vi "Get Sub Items.vi"(8 "error in (no error)":errorcluster, 11 "Type in":variant) -> (0 "error out":errorcluster, 2 "Sub Items":cluster{"Sub Items":T1[]}[](array[cluster]), 3 "Type out":variant)   [LabVIEW 2015, in "Read-Write-Signals.xnode"]
uses:
  Read-Write-Signals.xnode
  Read-Write-Signals Sub Item.ctl
  Read-Write-Signals Sub Item Type.ctl
  <vilib>/Utility/Data Type/NI_Data Type.lvlib
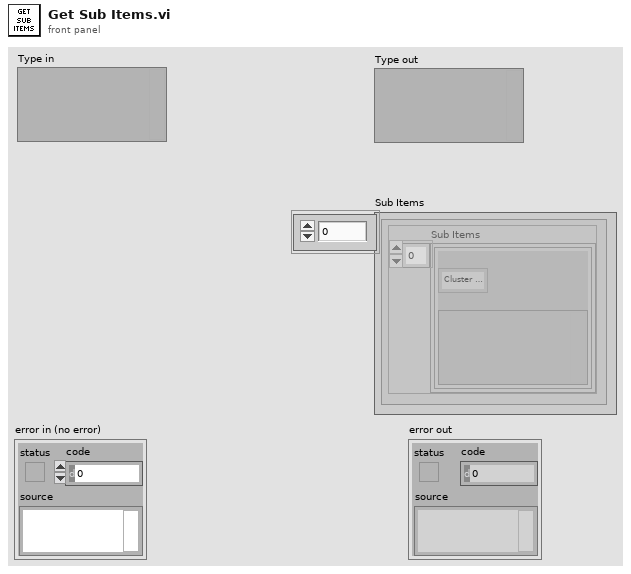
[diagram p1: front panel]
types:
  T1 = typedef "Read-Write-Signals Sub Item.ctl" = cluster{"Type":T2, "Value":variant}
  T2 = typedef "Read-Write-Signals Sub Item Type.ctl" = enum8{"Cluster Element", "Array Element", "Subarray"}
  T3 = typedef "NI_Data Type.lvlib/Data Type.ctl" = enum8{"Invalid Type", "Void", "I8", "I16", "I32", "I64", "U8", "U16", "U32", "U64", "Single Float", "Double Float", "Extended Float", "Single Complex", "Double Complex", "Extended Complex", "Enum U8", "Enum U16", "Enum U32", "Enum U64", "Single Float With Unit", "Double Float With Unit", "Extended Float With Unit", "Single Complex with Unit", "Double Complex with Unit", "Extended Complex with Unit", "Boolean", "String", "Path", "Picture", "Tag", "Array", "Cluster", "Variant", "LV Variant", "Waveform", "Timestamp", "Digital Waveform", "Digital Data", "ExpressData", "Refnum", "External Data", "VI", "Poly VI", "LabVIEW Class Instance", "Fixed Point"}
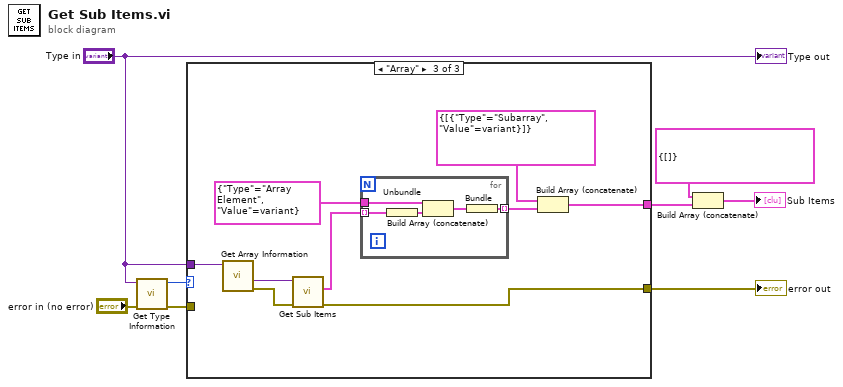
[diagram p0: block diagram]
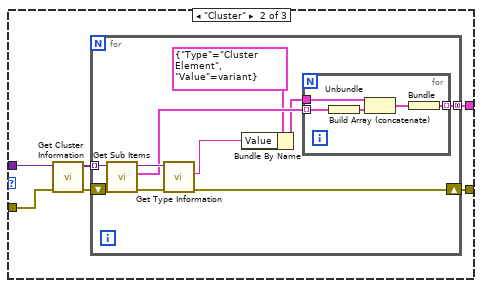
[diagram p3: hidden frame]
diagram:
  n1 = call <vilib>:"Get Type Information.vi"("error in (no error)"="error in (no error)", "Variant"="Type in") -> ("error out"=w6:errorcluster, "Type"=w8:T3)  [unwired: 5 in, 3 out]
  n2 = case shown="\"Array\"" w8 {
    tunnel: "Type in" -> [_ w15 w38]
    tunnel: w6 -> [w9 w14 _]
    tunnel: [_ w11 w31] -> w3
    tunnel: [w9 w10 w35] -> w4
    frame Default {
    }
    frame "Cluster" {
      n3 = call <vilib>:"Get Cluster Information.vi"("error in (no error)"=w14, "Variant"=w15) -> ("error out"=w12:errorcluster, "Cluster Elements"=w13:variant[])  [unwired: 8 in]
      n4 = for {
        tunnel: w13 -> [w25] mode=indexing
        tunnel: [w17] -> w11 mode=concatenating
        shift-right: [w16] -> w10
        shift-left: w12 -> [w24]
        n5 = call "Get Sub Items.vi"("error in (no error)"=w24, "Type in"=w25) -> ("error out"=w22:errorcluster, "Sub Items"=w21:cluster{"Sub Items":T1[]}[], "Type out"=w23:variant)  [unwired: 7 in]
        n6 = call <vilib>:"Get Type Information.vi"("error in (no error)"=w22, "Variant"=w23) -> ("error out"=w16:errorcluster, "Name"=w19:string)  [unwired: 5 in, 3 out]
        n7 = Bundle By Name(cluster=T1 {"Type"=enum."Cluster Element", "Value"=variant} ("Sub Items 2"), "Value"=w19) -> (w18:T1)
        n8 = for {
          tunnel: w21 -> [w30] mode=indexing
          tunnel: w18 -> [w28]
          tunnel: [w26] -> w17 mode=indexing
          n9 = Unbundle(w30) -> ("Sub Items"=w29:T1[])
          n10 = Build Array (concatenate)(w28, w29) -> (w27:T1[])
          n11 = Bundle(w27) -> (w26:cluster{T1[]})  [unwired: 1 in]
        }
      }
    }
    frame "Array" {
      n12 = call <vilib>:"Get Array Information.vi"("Variant"=w38) -> ("error out"=w36:errorcluster, "Array Element Data Type"=w37:variant)  [unwired: 7 in, 2 out]
      n13 = call "Get Sub Items.vi"("error in (no error)"=w36, "Type in"=w37) -> ("error out"=w35:errorcluster, "Sub Items"=w39:cluster{"Sub Items":T1[]}[])  [unwired: 7 in, 1 out]
      n14 = for {
        tunnel: w39 -> [w44] mode=indexing
        tunnel: T1 {"Type"=enum."Array Element", "Value"=variant} ("Sub Items 2") -> [w42]
        tunnel: [w40] -> w33 mode=indexing
        n15 = Unbundle(w44) -> ("Sub Items"=w43:T1[])
        n16 = Build Array (concatenate)(w42, w43) -> (w41:T1[])
        n17 = Bundle(w41) -> (w40:cluster{T1[]})  [unwired: 1 in]
      }
      n18 = Build Array (concatenate)(cluster{T1[]} {[{"Type"=enum."Subarray", "Value"=variant}]}, w33) -> (w31:cluster{T1[]}[])
    }
  }
  "error out" <- w4
  n19 = Build Array (concatenate)(cluster{T1[]} {[]}, w3) -> (→"Sub Items":cluster{T1[]}[])
  "Type out" <- "Type in"
